vi "write_sub_pend.vi"(0 "instance":i32, 1 "Enable Motor":bool, 7 "direction":dbl, 11 "motorEffort":i32) -> ()   [LabVIEW 2025]
uses:
  SADI_Pendulum_lib/pendulumApp.lvlib
panel:
  out "function return":i32
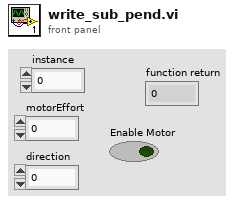
[diagram p1: front panel]
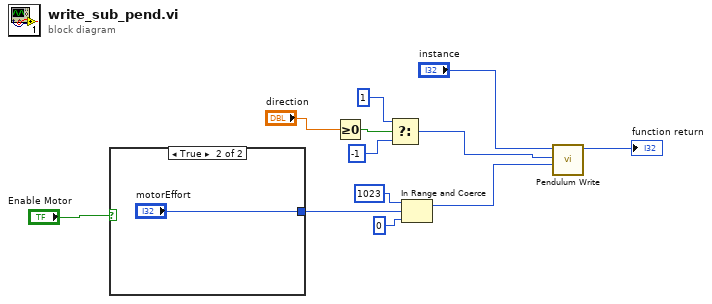
[diagram p0: block diagram]
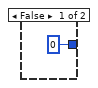
[diagram p2: hidden frame]
diagram:
  n1 = case shown="True" "Enable Motor" {
    tunnel: [0 ("motorEffort") "motorEffort"] -> w10
    frame False {
    }
    frame True {
    }
  }
  n2 = Greater Or Equal To 0?(x="direction") -> (x >= 0?=w2:bool)
  n3 = Select(t=1, s=w2, f=-1) -> (s? t:f=w4:i32)
  n4 = In Range and Coerce(upper limit=1023, x=w10, lower limit=0) -> (coerced(x)=w9:i32)  [unwired: 1 out]
  n5 = call "Pendulum Write.vi"("motorEffort"=w9, "direction"=w4, "instance"="instance") -> ("function return"=→"function return":i32)  [unwired: 8 in]
